vi "matrix_operations.vi"() -> ()   [LabVIEW 2016]
doc: "Shows the fundamental behavior and functionality of the matrix data type. While the test is running, you can change the matrix inputs or select built-in or user-defined numeric operations. Change the operation mode between matrix and array versions of the operations to see the difference in results."
uses:
  <vilib>/Analysis/Matrix/Datatypes/RealMatrix.ctl
  <vilib>/Analysis/Matrix/Datatypes/ComplexMatrix.ctl
  <vilib>/Analysis/Matrix/Numeric/Add/Add - RM,RM.vi
  <vilib>/Analysis/Matrix/Numeric/Conversions/Matrix To Array - RM.vi
  <vilib>/Analysis/Matrix/Numeric/Conversions/Array To Matrix - RA2.vi
  <vilib>/Analysis/Matrix/Numeric/Multiply/Multiply - RM,RM.vi
  <vilib>/Analysis/Matrix/Numeric/Exponential/Exponential - RM.vi
  <vilib>/Analysis/Matrix/Numeric/Natural Logarithm/Natural Logarithm - RM.vi
  <vilib>/Analysis/Matrix/Numeric/Square Root/Square Root - RM.vi
  <vilib>/Analysis/Matrix/Numeric/Conversions/Array To Matrix - CA2.vi
  <vilib>/Analysis/Matrix/Numeric/Complex/Cartesian To Complex - RM,RM.vi
  <vilib>/Analysis/Matrix/Numeric/Conversions/Array To Matrix - RA.vi
  <vilib>/Analysis/Matrix/NI_Matrix.lvlib
panel:
  in  "Mode":u16(ring) items=["Array", "Matrix"]
  in  "Real Matrix B":T1=[[1.0, 2.0], [3.0, 4.0]]
  out "Complex Matrix Result":T2
  out "Real Matrix Result":T1
  in  "Operation":u16(ring) items=["Decrement", "Add", "Multiply", "Exponential", "Natural Logarithm", "Square Root", "Cartesian To Complex", "Add Identity", "Sum Columns"]
  in  "Real Matrix A":T1=[[1.0, 0.0], [1.0, 1.0]]
  # "Overview: Demonstrates the fundamental behavior and functionality of the Matrix data type.\nRequirements: LabVIEW Full Development System\nInstructions: \n1. Run the VI.\n2. Modify the Real Matrix inputs, Operation and Mode, and view the Real Matrix Result.\n3. Click Stop to stop the VI."
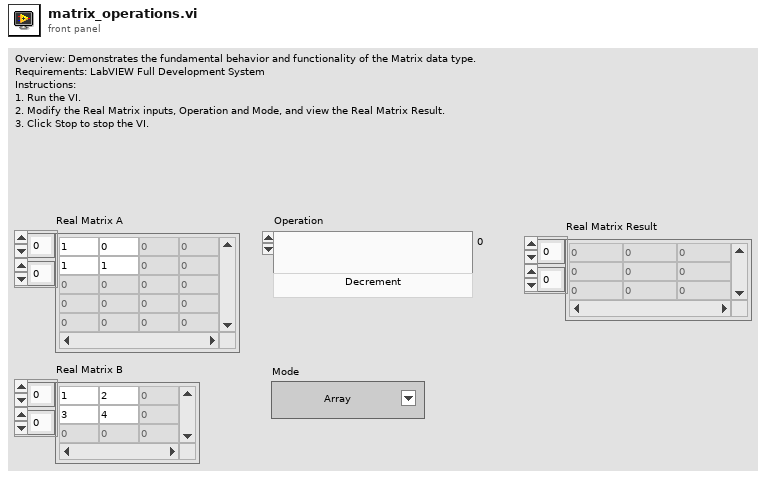
[diagram p1: front panel]
types:
  T1 = typedef "NI_Matrix.lvlib/RealMatrix.ctl" = dbl[][]
  T2 = typedef "NI_Matrix.lvlib/ComplexMatrix.ctl" = cdb[][]
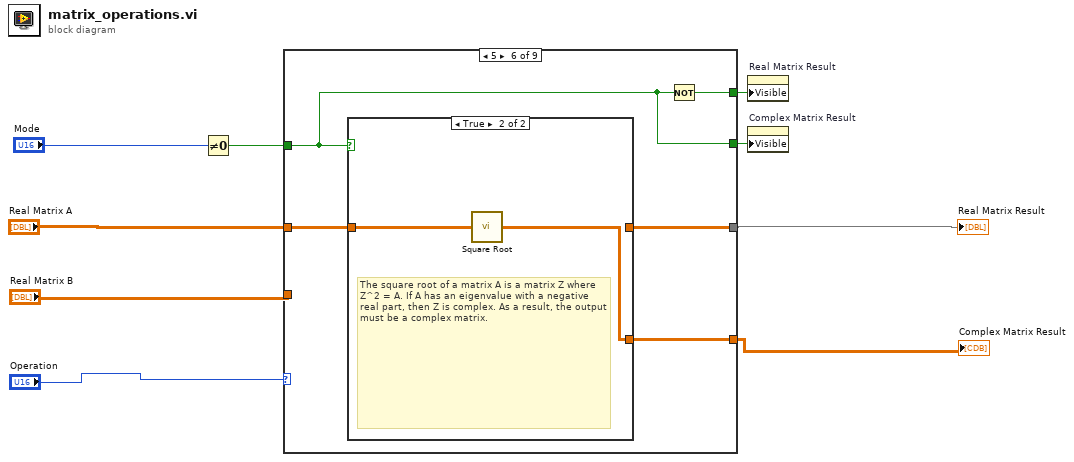
[diagram p0: block diagram]
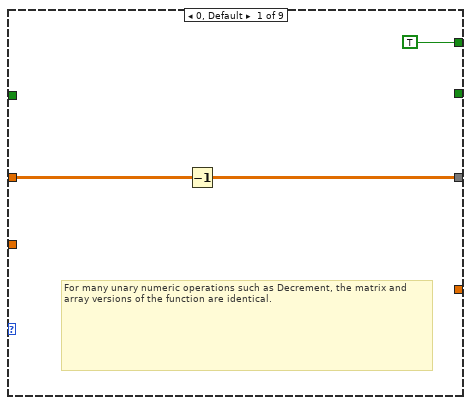
[diagram p2: hidden frame]
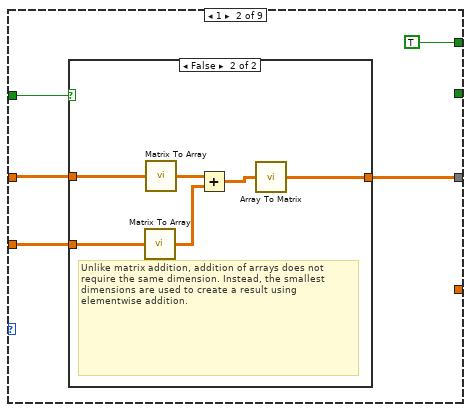
[diagram p3: hidden frame]
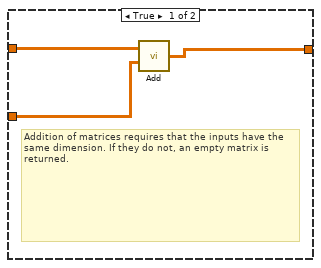
[diagram p4: hidden frame]
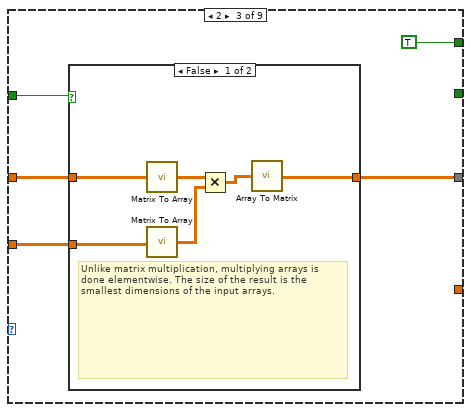
[diagram p5: hidden frame]
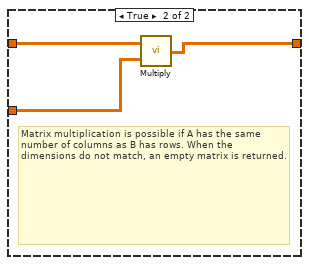
[diagram p6: hidden frame]
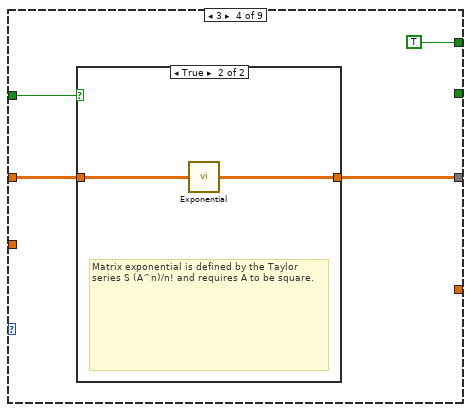
[diagram p7: hidden frame]
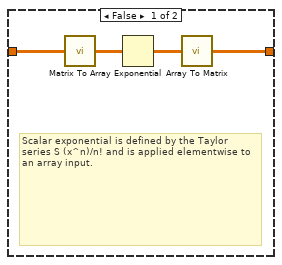
[diagram p8: hidden frame]
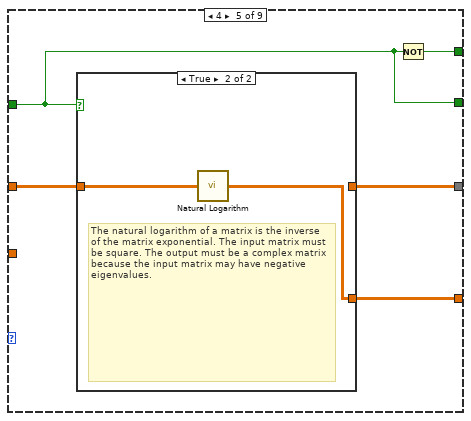
[diagram p9: hidden frame]
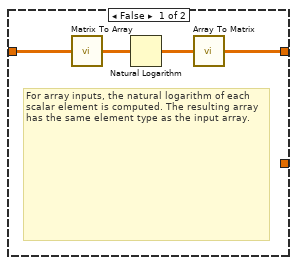
[diagram p10: hidden frame]
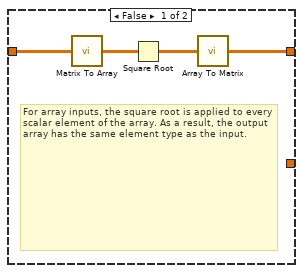
[diagram p11: hidden frame]
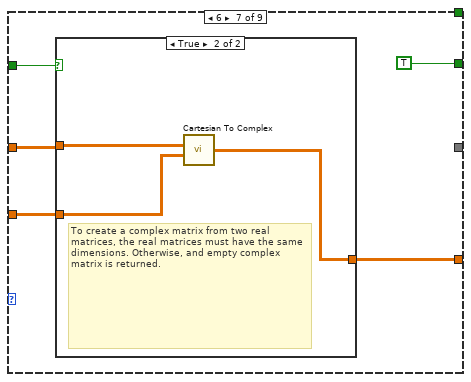
[diagram p12: hidden frame]
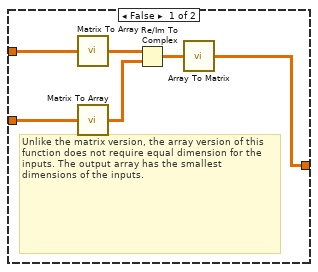
[diagram p13: hidden frame]
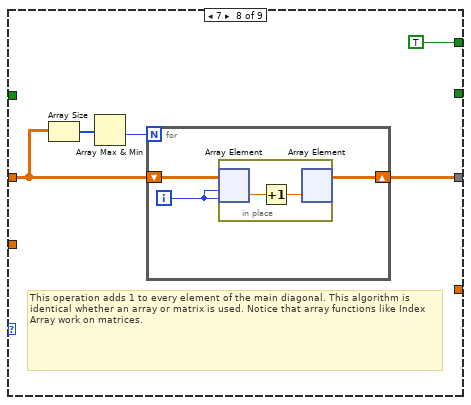
[diagram p14: hidden frame]
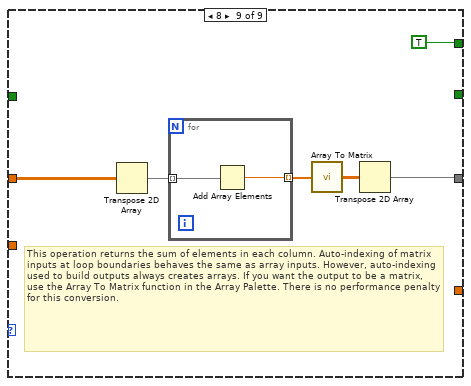
[diagram p15: hidden frame]
diagram:
  n1 = Not Equal To 0?(x="Mode") -> (x != 0?=w9:bool)
  n2 = case shown="5" "Operation" {
    tunnel: "Real Matrix A" -> [w12 w17 w31 w43 w55 w66 w77 w89 w102]
    tunnel: [w11 w15 w29 w44 w53 w64 _ w87 w98] -> w6
    tunnel: "Real Matrix B" -> [_ w16 w30 _ _ _ w76 _ _]
    tunnel: [_ _ _ _ w54 w65 w75 _ _] -> w5
    tunnel: w9 -> [_ w14 w27 w41 w51 w62 w73 _ _]
    tunnel: [TRUE TRUE TRUE TRUE w52 w63 _ TRUE TRUE] -> w7
    tunnel: [_ _ _ _ w51 w62 TRUE _ _] -> w8
    frame 0, Default {
      # "For many unary numeric operations such as Decrement, the matrix and array versions of the function are identical."
      n3 = Decrement(x=w12) -> (x-1=w11:T1)
    }
    frame 1 {
      n4 = case shown="False" w14 {
        tunnel: w17 -> [w20 w26]
        tunnel: w16 -> [w19 w25]
        tunnel: [w18 w21] -> w15
        frame True {
          # "Addition of matrices requires that the inputs have the same dimension. If they do not, an empty matrix is returned."
          n5 = call-poly <vilib>:"Add.vi"("Real Matrix B"=w19, "Real Matrix A"=w20) -> ("A + B"=w18:T1)
        }
        frame False {
          # "Unlike matrix addition, addition of arrays does not require the same dimension. Instead, the smallest dimensions are used to create a result using elementwise addition."
          n6 = call-poly <vilib>:"Matrix To Array.vi"("Real Matrix"=w25) -> ("Real 2D Array"=w22:dbl[][])
          n7 = call-poly <vilib>:"Matrix To Array.vi"("Real Matrix"=w26) -> ("Real 2D Array"=w23:dbl[][])
          n8 = Add ("Add.vi")(x=w23, y=w22) -> (x+y=w24:dbl[][])
          n9 = call-poly <vilib>:"Array To Matrix.vi"("Real 2D Array"=w24) -> ("Real Matrix"=w21:T1)
        }
      }
    }
    frame 2 {
      n10 = case shown="False" w27 {
        tunnel: w31 -> [w34 w40]
        tunnel: w30 -> [w33 w39]
        tunnel: [w37 w38] -> w29
        frame False {
          # "Unlike matrix multiplication, multiplying arrays is done elementwise. The size of the result is the smallest dimensions of the input arrays."
          n11 = call-poly <vilib>:"Matrix To Array.vi"("Real Matrix"=w34) -> ("Real 2D Array"=w35:dbl[][])
          n12 = call-poly <vilib>:"Matrix To Array.vi"("Real Matrix"=w33) -> ("Real 2D Array"=w32:dbl[][])
          n13 = Multiply(x=w35, y=w32) -> (x*y=w36:dbl[][])
          n14 = call-poly <vilib>:"Array To Matrix.vi"("Real 2D Array"=w36) -> ("Real Matrix"=w37:T1)
        }
        frame True {
          # "Matrix multiplication is possible if A has the same number of columns as B has rows. When the dimensions do not match, an empty matrix is returned."
          n15 = call-poly <vilib>:"Multiply.vi"("Real Matrix B"=w39, "Real Matrix A"=w40) -> ("A * B"=w38:T1)
        }
      }
    }
    frame 3 {
      n16 = case shown="True" w41 {
        tunnel: [w46 w50] -> w44
        tunnel: w43 -> [w48 w49]
        frame False {
          # "Scalar exponential is defined by the Taylor series S (x^n)/n! and is applied elementwise to an array input."
          n17 = call-poly <vilib>:"Matrix To Array.vi"("Real Matrix"=w48) -> ("Real 2D Array"=w47:dbl[][])
          n18 = Exponential ("Exponential.vi")(1:w47) -> (0:w45:dbl[][])
          n19 = call-poly <vilib>:"Array To Matrix.vi"("Real 2D Array"=w45) -> ("Real Matrix"=w46:T1)
        }
        frame True {
          # "Matrix exponential is defined by the Taylor series S (A^n)/n! and requires A to be square."
          n20 = call-poly <vilib>:"Exponential.vi"("Real Matrix A"=w49) -> ("e^A"=w50:T1)
        }
      }
    }
    frame 4 {
      n21 = case shown="True" w51 {
        tunnel: w55 -> [w57 w61]
        tunnel: [_ w60] -> w54
        tunnel: [w56 _] -> w53
        frame False {
          # "For array inputs, the natural logarithm of each scalar element is computed. The resulting array has the same element type as the input array."
          n22 = call-poly <vilib>:"Matrix To Array.vi"("Real Matrix"=w57) -> ("Real 2D Array"=w58:dbl[][])
          n23 = Natural Logarithm ("Natural Logarithm.vi")(1:w58) -> (0:w59:dbl[][])
          n24 = call-poly <vilib>:"Array To Matrix.vi"("Real 2D Array"=w59) -> ("Real Matrix"=w56:T1)
        }
        frame True {
          # "The natural logarithm of a matrix is the inverse  of the matrix exponential. The input matrix must be square. The output must be a complex matrix because the input matrix may have negative eigenvalues."
          n25 = call-poly <vilib>:"Natural Logarithm.vi"("Real Matrix A"=w61) -> ("ln(A)"=w60:T2)
        }
      }
      n26 = Not(x=w51) -> (.not. x?=w52:bool)
    }
    frame 5 {
      n27 = case shown="True" w62 {
        tunnel: w66 -> [w70 w72]
        tunnel: [_ w71] -> w65
        tunnel: [w67 _] -> w64
        frame False {
          # "For array inputs, the square root is applied to every scalar element of the array. As a result, the output array has the same element type as the input."
          n28 = call-poly <vilib>:"Matrix To Array.vi"("Real Matrix"=w70) -> ("Real 2D Array"=w69:dbl[][])
          n29 = Square Root ("Square Root.vi")(x=w69) -> (sqrt(x)=w68:dbl[][])
          n30 = call-poly <vilib>:"Array To Matrix.vi"("Real 2D Array"=w68) -> ("Real Matrix"=w67:T1)
        }
        frame True {
          # "The square root of a matrix A is a matrix Z where Z^2 = A. If A has an eigenvalue with a negative real part, then Z is complex. As a result, the output must be a complex matrix."
          n31 = call-poly <vilib>:"Square Root.vi"("Real Matrix A"=w72) -> ("sqrt(A)"=w71:T2)
        }
      }
      n32 = Not(x=w62) -> (.not. x?=w63:bool)
    }
    frame 6 {
      n33 = case shown="True" w73 {
        tunnel: w77 -> [w82 w86]
        tunnel: w76 -> [w83 w85]
        tunnel: [w78 w84] -> w75
        frame False {
          # "Unlike the matrix version, the array version of this function does not require equal dimension for the inputs. The output array has the smallest dimensions of the inputs."
          n34 = call-poly <vilib>:"Matrix To Array.vi"("Real Matrix"=w82) -> ("Real 2D Array"=w81:dbl[][])
          n35 = call-poly <vilib>:"Matrix To Array.vi"("Real Matrix"=w83) -> ("Real 2D Array"=w80:dbl[][])
          n36 = Re/Im To Complex ("Cartesian To Complex.vi")(1:w80, 2:w81) -> (0:w79:cdb[][])
          n37 = call-poly <vilib>:"Array To Matrix.vi"("Complex 2D Array"=w79) -> ("Complex Matrix"=w78:T2)
        }
        frame True {
          # "To create a complex matrix from two real matrices, the real matrices must have the same dimensions. Otherwise, and empty complex matrix is returned."
          n38 = call-poly <vilib>:"Cartesian To Complex.vi"("Real Matrix I"=w85, "Real Matrix R"=w86) -> ("R + Ii"=w84:T2)
        }
      }
    }
    frame 7 {
      # "This operation adds 1 to every element of the main diagonal. This algorithm is identical whether an array or matrix is used. Notice that array functions like Index Array work on matrices."
      n39 = Array Size(array=w89) -> (size(s)=w90:i32[])
      n40 = Array Max & Min(array=w90) -> (min value=w88:i32)  [unwired: 3 out]
      n41 = for {
        N: w88 -> [_]
        shift-right: [w93] -> w87
        shift-left: w89 -> [w94]
        i -> [w92]
        n42 = in-place {
          n43 = in-place-array #1(w94, w92, w92) -> (w96:dbl)
          n44 = Increment(x=w96) -> (x+1=w95:dbl)
          n45 = in-place-array #1(w95) -> (w93:T1)  [unwired: 2 out]
        }
      }
    }
    frame 8 {
      # "This operation returns the sum of elements in each column. Auto-indexing of matrix inputs at loop boundaries behaves the same as array inputs. However, auto-indexing used to build outputs always creates arrays. If you want the output to be a matrix, use the Array To Matrix function in the Array Palette. There is no performance penalty for this conversion."
      n46 = Transpose 2D Array(2D array=w102) -> (transposed array=w101:T1)
      n47 = for {
        tunnel: w101 -> [w104] mode=indexing
        tunnel: [w103] -> w100 mode=indexing
        n48 = Add Array Elements(numeric array=w104) -> (sum=w103:dbl)
      }
      n49 = call-poly <vilib>:"Array To Matrix.vi"("Real 1D Array"=w100) -> ("Real Matrix (Column Vector)"=w99:T1)
      n50 = Transpose 2D Array(2D array=w99) -> (transposed array=w98:T1)
    }
  }
  "Complex Matrix Result" <- w5
  "Real Matrix Result" <- w6
  n51 = property on="Real Matrix Result" class="Arr (strict)"("Visible"=w7) -> ()  [unwired: 2 in, 2 out]
  n52 = property on="Complex Matrix Result" class="Arr (strict)"("Visible"=w8) -> ()  [unwired: 2 in, 2 out]
